vi "XML_EEG_hexStringToWaveform.vi"(8 "error in (no error)":errorcluster, 11 "Hex String in":string) -> (0 "error out":errorcluster, 3 "Waveform out":waveform(dbl))   [LabVIEW 2016, in "XML_EEG_File_Parser.lvlib"]
uses:
  XML_EEG_File_Parser.lvlib
panel:
  # "This VI is a part of BCI Design library, http://www.ru-bci.org \nCopyright © 2020, Sotnikov Peter, All rights reserved. License: GNU GPLv3"
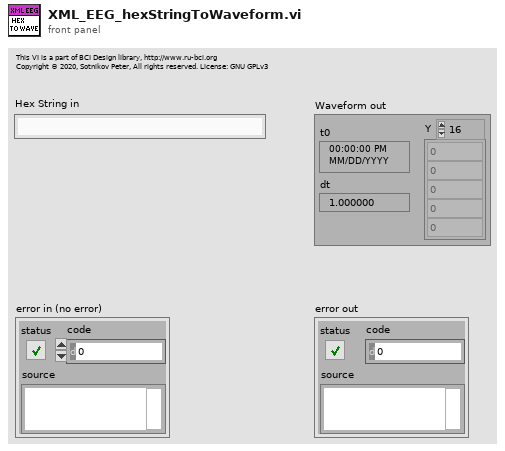
[diagram p1: front panel]
types:
  T1 = enum16{"big-endian, network order", "native, host order", "little-endian"}
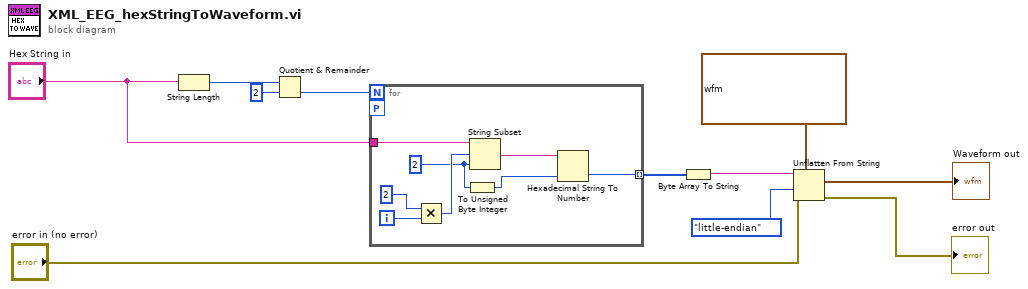
[diagram p0: block diagram]
diagram:
  n1 = String Length(string="Hex String in") -> (length=w11:i32)
  n2 = Quotient & Remainder(x=w11, y=2) -> (floor(x/y)=w9:i32)  [unwired: 1 out]
  n3 = for {
    N: w9 -> [_]
    tunnel: "Hex String in" -> [w19]
    tunnel: [w12] -> w7 mode=indexing
    workers-P: _ -> [_]
    i -> [w18]
    w14 = 2 ("length (rest)")
    n4 = Multiply(x=2, y=w18) -> (x*y=w16:i32)
    n5 = To Unsigned Byte Integer(number=w14) -> (unsigned 8bit integer=w15:u8)
    n6 = String Subset(string=w19, offset (0)=w16, length (rest)=w14) -> (substring=w13:string)
    n7 = Hexadecimal String To Number(string=w13, default (0uL)=w15) -> (number=w12:u8)  [unwired: 1 in, 1 out]
  }
  n8 = Byte Array To String(unsigned byte array=w7) -> (string=w6:string)
  n9 = Unflatten From String(type=waveform(dbl) {"t0"=timestamp(0 s since 1904-01-01), "dt"=1.0, "Y"=[]} ("Waveform"), binary string=w6, byte order (0:big-endian, network order)=T1."little-endian", error in (no error)="error in (no error)") -> (value=→"Waveform out":waveform(dbl), error out=→"error out":errorcluster)  [unwired: 1 in, 1 out]
